vi "init.vi"(8 "error in (no error)":errorcluster, 11 "ForceSensor in":refnum<class "ForceSensor.lvclass">) -> (0 "error out":errorcluster, 3 "ForceSensor out":refnum<class "ForceSensor.lvclass">)   [LabVIEW 2013, in "ForceSensor.lvclass"]
uses:
  ForceSensor.lvclass
  Configuration/Force Sensor.ctl
  ForceSensor.lvclass/ForceSensor.ctl
  ConfigurationThisComponent/ConfigurationThisComponent.lvclass
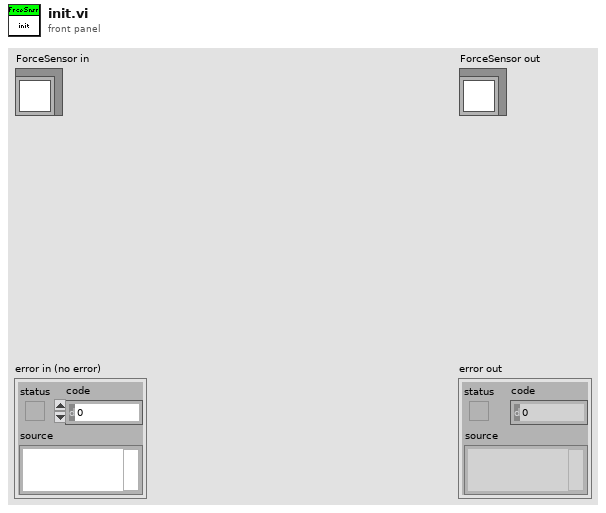
[diagram p1: front panel]
types:
  T1 = typedef "Force Sensor.ctl" = cluster{"Force Sensor Conversion":dbl[unit]}
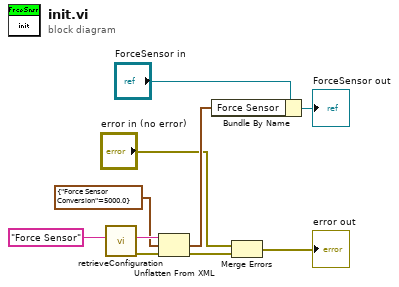
[diagram p0: block diagram]
diagram:
  n1 = call "retrieveConfiguration.vi"("configName"="Force Sensor") -> ("error out"=w7:errorcluster, "xmlConfig"=w5:string)  [unwired: 8 in, 1 out]
  n2 = Unflatten From XML(xml string=w5, type=T1 {"Force Sensor Conversion"=5000.0} ("Force Sensor"), error in (no error)=w7) -> (value=w10:T1, error out=w9:errorcluster)
  n3 = Bundle By Name(cluster="ForceSensor in", "Force Sensor"=w10) -> (→"ForceSensor out":refnum<class "ForceSensor.lvclass">)
  n4 = Merge Errors("error in (no error)", w9) -> (→"error out":errorcluster)
